vi "Gas to File Gas ID.vi"(11 "Gas":string) -> (3 "gasID":i32)   [LabVIEW 2015]
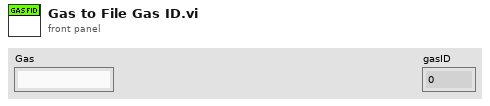
[diagram p1: front panel]
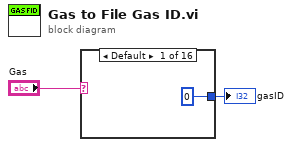
[diagram p0: block diagram]
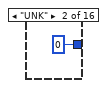
[diagram p2: hidden frame]
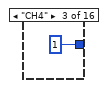
[diagram p3: hidden frame]
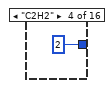
[diagram p4: hidden frame]
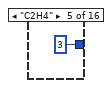
[diagram p5: hidden frame]
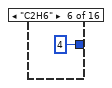
[diagram p6: hidden frame]
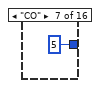
[diagram p7: hidden frame]
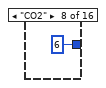
[diagram p8: hidden frame]
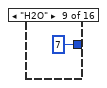
[diagram p9: hidden frame]
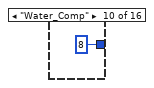
[diagram p10: hidden frame]
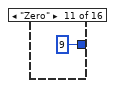
[diagram p11: hidden frame]
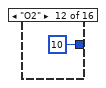
[diagram p12: hidden frame]
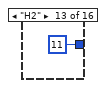
[diagram p13: hidden frame]
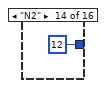
[diagram p14: hidden frame]
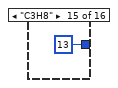
[diagram p15: hidden frame]
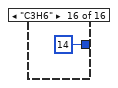
[diagram p16: hidden frame]
diagram:
  n1 = case shown="Default" "Gas" {
    tunnel: [0 ("gasID") 0 ("gasID") 1 ("gasID") 2 ("gasID") 3 ("gasID") 4 ("gasID") 5 ("gasID") 6 ("gasID") 7 ("gasID") 8 ("gasID") 9 ("gasID") 10 ("gasID") 11 ("gasID") 12 ("gasID") 13 ("gasID") 14 ("gasID")] -> w1
    frame Default {
    }
    frame "UNK" {
    }
    frame "CH4" {
    }
    frame "C2H2" {
    }
    frame "C2H4" {
    }
    frame "C2H6" {
    }
    frame "CO" {
    }
    frame "CO2" {
    }
    frame "H2O" {
    }
    frame "Water_Comp" {
    }
    frame "Zero" {
    }
    frame "O2" {
    }
    frame "H2" {
    }
    frame "N2" {
    }
    frame "C3H8" {
    }
    frame "C3H6" {
    }
  }
  "gasID" <- w1
